vi "test Segmented Upload Visible String C5-E.vi"(11 "Test Case In":refnum<class "Tests SDO Manager.lvclass">) -> (0 "error out":errorcluster, 3 "Test Case Out":refnum<class "Tests SDO Manager.lvclass">)   [LabVIEW 2020, in "Tests SDO Manager.lvclass"]
uses:
  Tests SDO Manager.lvclass
  Tests SDO Manager.lvclass/Tests SDO Manager.ctl
  HAL/HAL-Devices/source/PCAN USB Dongle/PCAN Basic 4/Configure Strategies/Read-Write CAN Frame Strategy/PCAN Basic4 Read-Write CAN CC Frame Strategy.lvclass
  D:/git/HAL/HAL-Devices/source/PCAN USB Dongle/PCAN Basic 4/Configure Strategies/Base Configure Strategy/PCAN Basic4 Base Configure Strategy.lvclass
  D:/git/HAL/Source/Interfaces/IApplyConfiguration/IApplyConfiguration.lvclass
  D:/git/HAL/Source/Interfaces/IClose/IClose.lvclass
  D:/git/HAL/Source/Interfaces/IInitialize/IInitialize.lvclass
  D:/git/HAL/Source/Interfaces/ICommunicate/ICommunicate.lvclass
  D:/git/HAL/Source/Interfaces/IRunnable/IRunnable.lvclass
  D:/git/HAL/Source/Interfaces/IValidate Configuration/IValidate Configuration.lvclass
  D:/git/HAL/HAL-Devices/source/PCAN USB Dongle/PCAN Basic 4/Configure Strategies/Read-Write CAN Frame Strategy/PCAN Basic4 Read-Write CAN CC Frame Strategy.lvclass
  HAL/Source/Communicator/Communicator.lvclass
  D:/git/HAL/Source/Interfaces/IInstrument/IInstrument.lvclass
  D:/git/HAL/Source/Communicator/Communicator.lvclass
  D:/git/HAL/Source/Interfaces/IConfigurable/IConfigurable.lvclass
  source/Logging/Logger/Logger.lvclass
  C:/Program Files/National Instruments/LabVIEW 2026/vi.lib/ActorFramework/Actor/Actor.lvclass
  D:/git/CANopen-LabVIEW/source/Logging/Logger/Logger.lvclass
  4993e8ee-a06a-463a-9684-69129f64d5ce.vi
  source/SDO Manager/SDO Manager/SDO Manager/SDO Manager.lvclass
  source/Logging/Log Level.vi
  source/Logging/CANopen Logging.lvlib
  <vilib>/ActorFramework/Actor/Actor.lvclass
  <vilib>/ActorFramework/Stop Msg/Stop Msg.lvclass
  source/SDO Manager/SDO Manager/SDO Manager/Upload Octet String.vi
  source/SDO Manager/SDO Manager/SDO Transfer/SDO abort code.ctl
  source/SDO Manager/SDO Manager/SDO Transfer/SDO Transfer.lvclass
  source/Typedefs/SDO Result.ctl
panel:
  out "Visible String":string
  out "SDO Result":T1={"Success"=FALSE, "SDO abort code"={"Null"=TRUE, "Value"=84082688}, "Data"={"Null"=TRUE, "Data"=[]}} {"SDO abort code"."Value" items=["Toggle bit not allowed"=84082688, "SDO protocol timed out"=84148224, "Client/server command specifier not valid or unknown"=84148225, "Invalid block size (block mode only)"=84148226, "Invalid sequence number (block mode only)"=84148227, "CRC error (block mode only)"=84148228, "Out of memory"=84148229, "Attempt to read a write only object"=100728833, "Attempt to write a read only object"=100728834, "Object does not exist in the object dictionary"=100794368, "Object cannot be mapped to the PDO"=100925505, "The number and length of the objects to be mapped would exceed PDO length"=100925506, "General parameter incompatibility reason"=100925507, "General internal incompatibility in the device"=100925511, "Access failed due to an hardware error"=101056512, "Data type does not match, length of service parameter does not match"=101122064, "Data type does not match, length of service parameter too high"=101122066, "Data type does not match, length of service parameter too low"=101122067, "Sub-index does not exist"=101253137, "Invalid value for parameter (download only)"=101253168, "Value of parameter written too high (download only)"=101253169, "Value of parameter written too low (download only)"=101253170, "Maximum value is less than minimum value"=101253174, "Resource not available: SDO connection"=101318691, "General error"=134217728, "Data cannot be transferred or stored to the application"=134217760, "Data cannot be transferred or stored to the application because of local control"=134217761, "Data cannot be transferred or stored to the application because of the present device stable"=134217762, "Object dictionary dynamic generation fails or no object dictionary is present (e.g. object dictionary is generated from file and generation fails because of an file error)"=134217763, "No data available"=134217764]; "Data"."Data" format="%02x"}
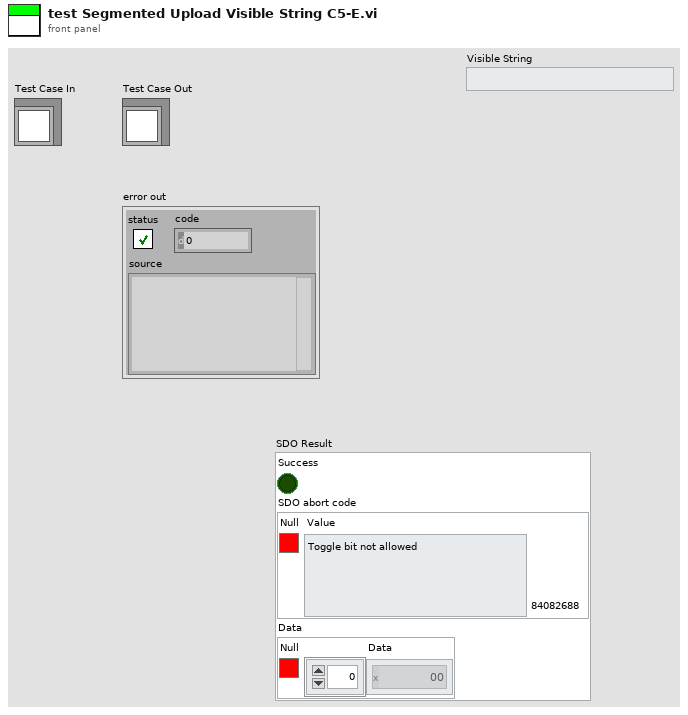
[diagram p1: front panel]
types:
  T1 = typedef "CANopen.lvlib/SDO Manager.lvlib/SDO Transfer.lvclass/SDO Result.ctl" = cluster{"Success":bool, "SDO abort code":cluster{"Null":bool, "Value":T2}, "Data":cluster{"Null":bool, "Data":u8[]}}
  T2 = typedef "CANopen.lvlib/SDO Manager.lvlib/SDO Transfer.lvclass/SDO abort code.ctl" = u32
  T3 = cluster{"Node-ID":u8, "Multiplexer":cluster{"Index":u16, "Sub-Index":u8}}
  T4 = enum16{"Error", "Warn", "Info", "Debug", "Trace"}
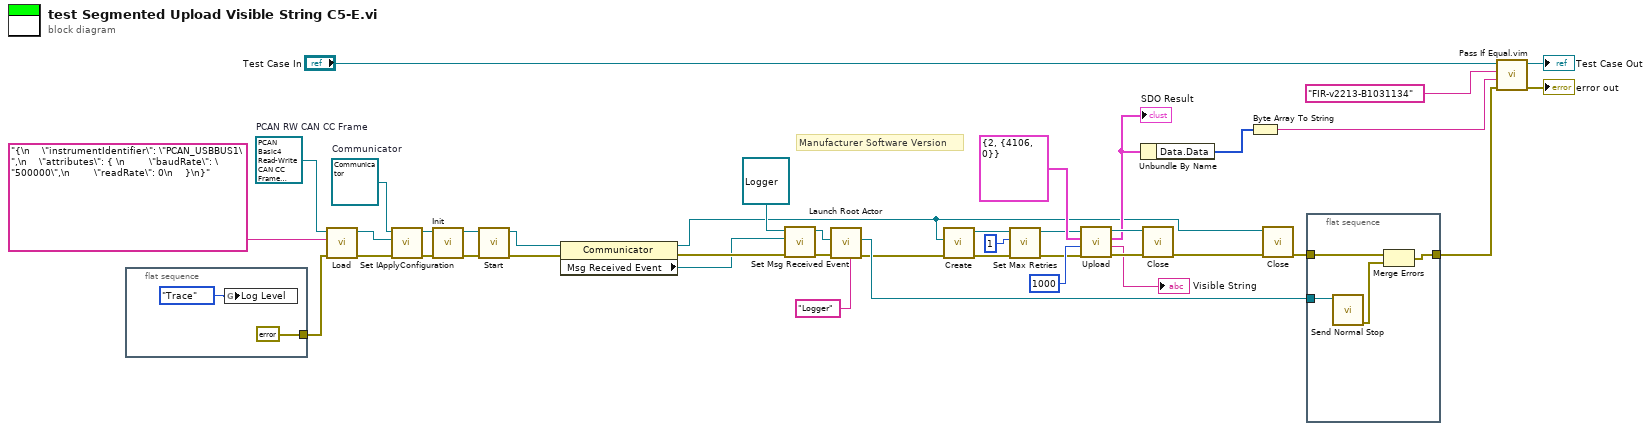
[diagram p0: block diagram]
diagram:
  w10 = refnum<class "Communicator.lvclass"> refnum  # Communicator
  w16 = refnum<class "PCAN Basic4 Read-Write CAN CC Frame Strategy.lvclass"> refnum  # PCAN RW CAN CC Frame
  # "Manufacturer Software Version"
  n1 = flat-sequence {
    tunnel: [errorcluster {"status"=FALSE, "code"=0, "source"=""} ("error constant")] -> w5
    frame #0 {
      n2 = global write "Log Level.vi" "Log Level"(T4."Trace" ("Log Level")) -> ()
    }
  }
  n3 = call-dynamic "Load.vi"("error in"=w5, "Source"="{\n    \"instrumentIdentifier\": \"PCAN_USBBUS1\",\n    \"attributes\": { \n        \"baudRate\": \"500000\",\n        \"readRate\": 0\n    }\n}", "PCAN Basic Base Configure Strategy in"=w16) -> ("error out"=w13:errorcluster, "PCAN Basic Base Configure Strategy out"=w14:refnum<class "PCAN Basic4 Read-Write CAN CC Frame Strategy.lvclass">)  [unwired: 7 in]
  n4 = call-dynamic "Set IApplyConfiguration.vi"("Error In"=w13, "IApplyConfiguration"=w14, "Communicator in"=w10) -> ("Error Out"=w12:errorcluster, "Communicator out"=w11:refnum<class "Communicator.lvclass">)  [unwired: 7 in]
  n5 = call-dynamic "Init.vi"("Error In"=w12, "Communicator in"=w11) -> ("Error Out"=w9:errorcluster, "Communicator out"=w8:refnum<class "Communicator.lvclass">)  [unwired: 8 in]
  n6 = call-dynamic "Start.vi"("Error In"=w9, "Communicator in"=w8) -> ("Error Out"=w7:errorcluster, "Communicator out"=w6:refnum<class "Communicator.lvclass">)  [unwired: 8 in]
  n7 = property class="Communicator"(reference=w6, error in=w7) -> (reference out=w18:refnum<class "Communicator.lvclass">, error out=w29:errorcluster, "Msg Received Event"=w1:refnum<user-event>)
  n8 = call "Set Msg Received Event.vi"("error in"=w29, "Msg Received Event"=w1, "Logger in"=refnum<class "Logger.lvclass"> refnum) -> ("error out"=w31:errorcluster, "Logger out"=w30:refnum<class "Logger.lvclass">)  [unwired: 7 in]
  n9 = call <vilib>:"Launch Root Actor.vi"("Debug Alias"="Logger", "error in (no error)"=w31, "Actor"=w30) -> ("error out"=w3:errorcluster, "Actor's Enqueuer"=w26:refnum<class "Message Enqueuer.lvclass">)  [unwired: 7 in]
  n10 = call "Create.vi"("Error In"=w3, "ICommunicate"=w18) -> ("Error Out"=w24:errorcluster, "SDO Manager"=w23:refnum<class "SDO Manager.lvclass">)  [unwired: 8 in]
  n11 = call "Set Max Retries.vi"("error in"=w24, "Max Retries"=u8 1, "SDO Manager in"=w23) -> ("error out"=w21:errorcluster, "SDO Manager out"=w22:refnum<class "SDO Manager.lvclass">)  [unwired: 7 in]
  n12 = call-poly "Upload.vi"("Error In"=w21, "Retry Delay (ms)"=1000 ("Timeout"), "Parameters"=T3 {"Node-ID"=2, "Multiplexer"={"Index"=4106, "Sub-Index"=0}}, "SDO Manager in"=w22) -> ("Error Out"=w36:errorcluster, "Octet String"=→"Visible String":string, "SDO Result"=w33:T1, "SDO Manager out"=w35:refnum<class "SDO Manager.lvclass">)  [unwired: 4 in]
  "SDO Result" <- w33
  n13 = Unbundle By Name(w33) -> ("Data.Data"=w32:u8[])
  n14 = call "Close.vi"("Error In"=w36, "SDO Manager"=w35) -> ("Error Out"=w38:errorcluster)  [unwired: 8 in, 1 out]
  n15 = Byte Array To String(unsigned byte array=w32) -> (string=w17:string)
  n16 = call-dynamic "Close.vi"("Error In"=w38, "Communicator in"=w18) -> ("Error Out"=w27:errorcluster)  [unwired: 8 in, 1 out]
  n17 = flat-sequence {
    tunnel: w27 -> [w44]
    tunnel: w26 -> [w47]
    tunnel: [w45] -> w25
    frame #0 {
      n18 = call <vilib>:"Send Normal Stop.vi"("Message Enqueuer"=w47) -> ("error out"=w46:errorcluster)  [unwired: 10 in]
      n19 = Merge Errors(w44, w46) -> (w45:errorcluster)
    }
  }
  n20 = call "Pass If Equal.vim"("error in (no error)"=w25, "Actual"=w17, "Expected"="FIR-v2213-B1031134", "LUnit Test Case In"="Test Case In") -> ("error out"=→"error out":errorcluster, "LUnit Test Case Out"=→"Test Case Out":refnum<class "Tests SDO Manager.lvclass">)  [unwired: 6 in]
